vi "Dymin_FPGA_Main.vi"() -> ()   [LabVIEW 2016]
doc: "This VI demonstrates how to use an external signal to control the execution rate of a while loop."
uses:
  <vilib>/Platform/TimedLoop/XDataNode/timing_clust.ctl
  <vilib>/Platform/TimedLoop/XDataNode/nitl_modes.ctl
  <vilib>/Platform/TimedLoop/XDataNode/wakeup.ctl
  <vilib>/rvi/Emulation/niFpgaGetClockAttributes.vi
  <vilib>/rvi/Emulation/niFpgaSctlEmulationGetInTimedLoop.vi
  <vilib>/rvi/Emulation/niFpgaEmulationReportErrorSimple.vi
  <vilib>/rvi/eio/common/nirviEmuTemplateMethod_errors.vi
  <vilib>/rvi/Emulation/niFpgaCriticalErrorInLSC.vi
  <vilib>/rvi/DataTransferAndStorage/Container/Common/niFpgaContainerExecOnDevCompGetState.vi
  <vilib>/rvi/Emulation/niFpgaEmulationIsFPGAContextNoSignature.vi
  <vilib>/rvi/errors/niFpgaSetErrorForExecOnDevCompSimple.vi
  <vilib>/rvi/eio/common/nirviEmuReportErrorAndStop.vi
  <vilib>/rvi/DataTransferAndStorage/Container/Common/niFpgaContainerGetUniqueNameForEmu.vi
  <vilib>/rvi/FIFO/Fifo_Resource/nirvififoEmulationSetSize.vi
  <vilib>/rvi/FIFO/Fifo_Resource/nirviFifoEmulationQueueMgr.vi
  <instcachedir>/0/nirviFifoEmulationQueueMgr_E5CAEC123FF24DC58D834DCA3CDAA9B5.lvgen/nirviFifoEmulationQueueMgr_E5CAEC123FF24DC58D834DCA3CDAA9B5_001.vi
  <vilib>/rvi/FIFO/Fifo_Resource/nirvififoEmulationDetermineInputValidOut.vi
  <vilib>/rvi/FIFO/Fifo_Resource/nirvififoEmulationCreateLock.vi
  <vilib>/rvi/Emulation/niFpgaProcessEmulError.vi
  <vilib>/rvi/FIFO/Fifo_Resource/nirvififoEmulationObtainLock.vi
  <vilib>/rvi/FIFO/Fifo_Resource/nirvififoEmulationReleaseLock.vi
  <vilib>/rvi/occurrence/nirviWaitOnOccurrenceBase.vi
  <vilib>/rvi/errors/nirviReportUnexpectedCaseInternalError.vi
  <vilib>/rvi/errors/nirviReportUnexpectedCaseInternalError (U32).vi
  <vilib>/Utility/error.llb/Clear Errors.vi
  <vilib>/rvi/interface/RandomDataEmulation/niFpgaRandomDataHandleErrors.vi
  <vilib>/eio/EIONode/EIONode.xnode
  <vilib>/Platform/TimedLoop/XDataNode/XDataNode.xnode
  <vilib>/rvi/DataTransferAndStorage/Container/XNode/niFpgaContainer.xnode
  <vilib>/rvi/FIFO/Fifo_Resource/niFpgaFifoEmulationRefIn.vi
  <vilib>/Platform/TimedLoop/XDataNode/XDNodeRunTimeDep.lvlib
panel:
  in  "Dymin On?":bool
  in  "stop 4":bool
  in  "stop 3":bool
  in  "stop 2":bool
  in  "stop":bool
  out "Index":i32
  out "Dymin Step":i32
  out "Counts":i32
  out "Last Index":i32
  out "Last Counts":i32
  in  "Time (#80MHz periods)":i32[](array[numeric])=[32, 32, 32, 32]
  in  "Threshold (counts)":i32[](array[numeric])=[0, 0, 0, 0]
  in  "AOM Volts":u16[](array[numeric])=[0, 82, 164, 246]
  # "12 bit ADC volts"
  # ".1=82\n.2=164\n.3=246"
  # "16=200ns\n32=400ns"
  # "0 value means the step before it was the last step"
  # "v5 new settings for multiplexer\nv6 new DIOs on 9/24/2020\nv7 new DIOs on 11/24/2020\nv8_2 Dymin on button"
  # "step with Time_i=0 is not done, last step must have a time and first step with time 0 is \nOR find another way to finish the Dymin, but for now do it this way."
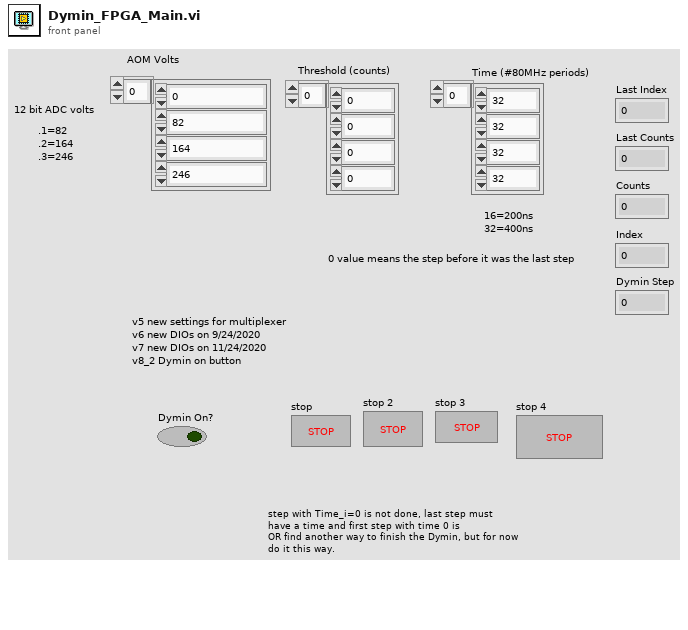
[diagram p1: front panel]
types:
  T1 = typedef "XDNodeRunTimeDep.lvlib/timing_clust.ctl" = cluster{"Expected End [f-1]":u64, "Actual End [f-1]":u64, "Finished Late? [f-1]":bool, "Expected End [i-1]":u64, "Actual End [i-1]":u64, "Finished Late? [i-1]":bool, "Expected Start [i]":u64, "Actual Start [i]":u64, "Expected Start [f]":u64, "Actual Start [f]":u64, "Source Name":string, "Structure Name":string, "Period":i64, "Deadline":i64, "Offset":i64, "Start":i64, "Priority":i32, "Timeout":i32, "Mode":T2, "Wakeup Reason":T3, "Error":errorcluster, "Source Type":string, "Secondary Source Type":string, "Global End Time":u64, "Global Start Time":u64, "Frame Duration":u64, "Iteration Duration":u64, "Assigned CPU":i32, "I/O Scan Engine Mode":u32}
  T2 = typedef "XDNodeRunTimeDep.lvlib/nitl_modes.ctl" = enum32{"No Change", "Process missed periods, maintain original phase", "Discard missed periods, maintain original phase", "Process missed periods, ignore original phase", "Discard missed periods, ignore original phase"}
  T3 = typedef "XDNodeRunTimeDep.lvlib/wakeup.ctl" = enum32{"Normal", "Aborted", "Asynchronous wakeup", "Timing source error", "Timed loop error", "Timeout"}
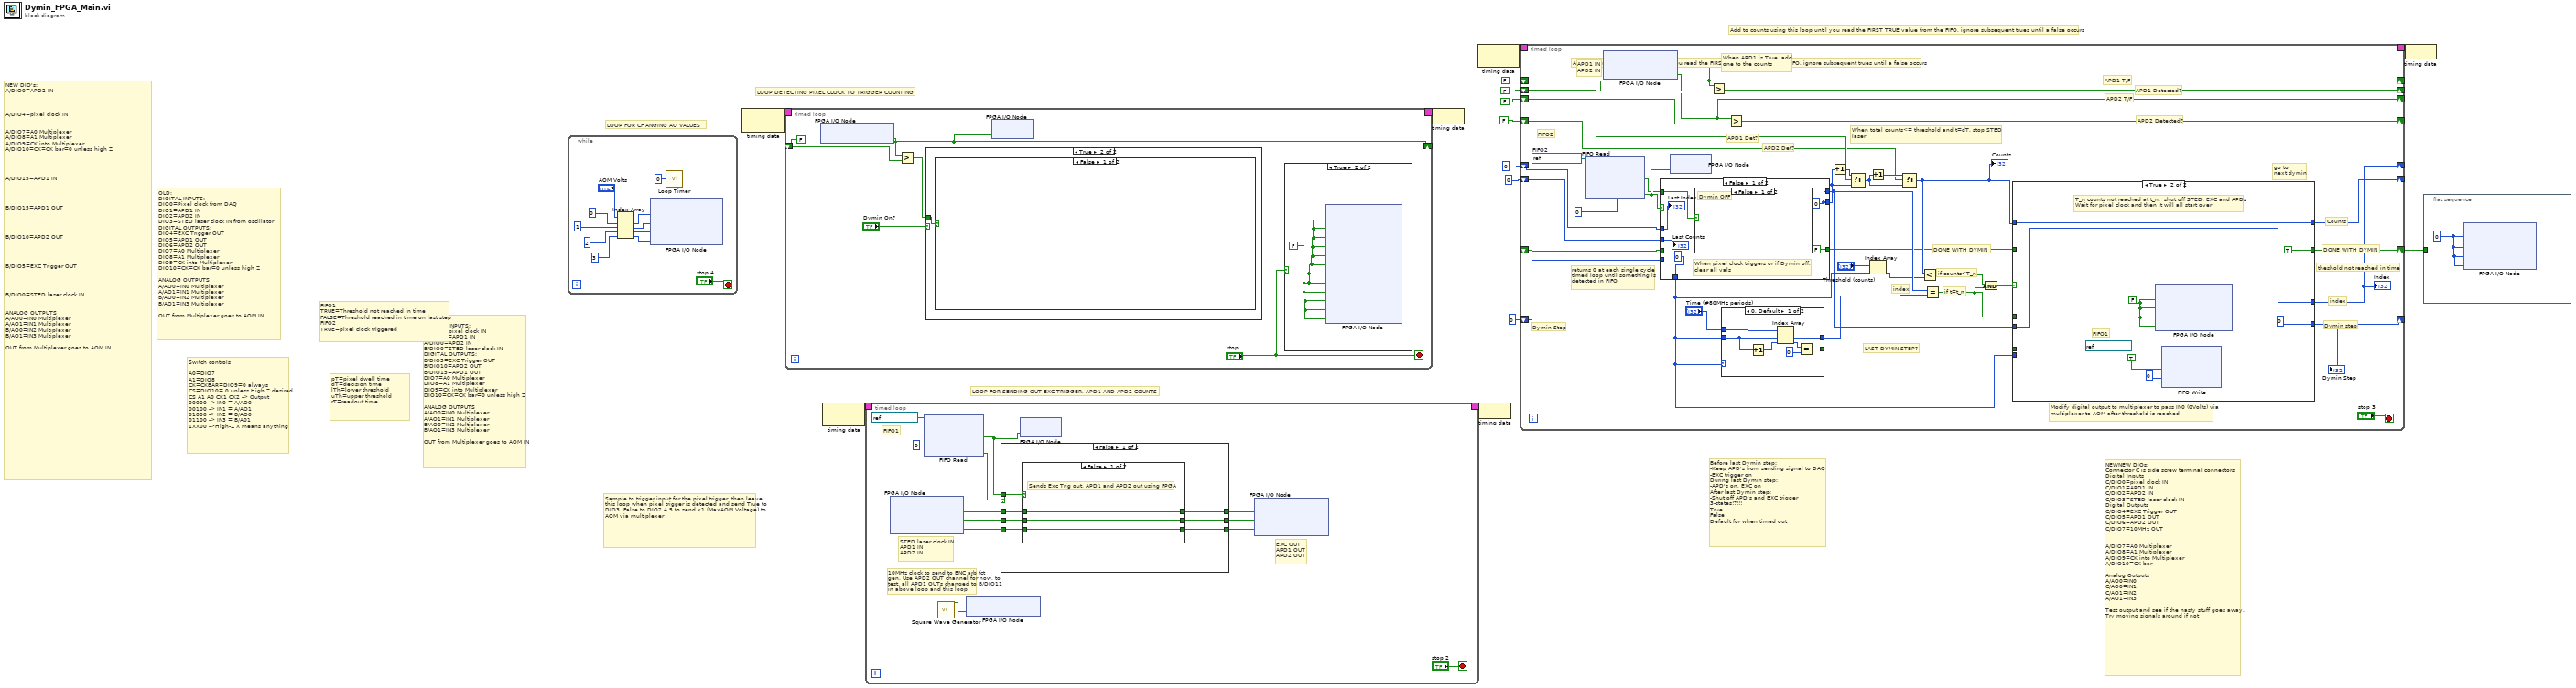
[diagram p0: block diagram]
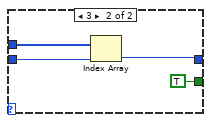
[diagram p2: hidden frame]
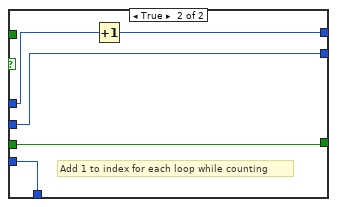
[diagram p4: hidden frame]
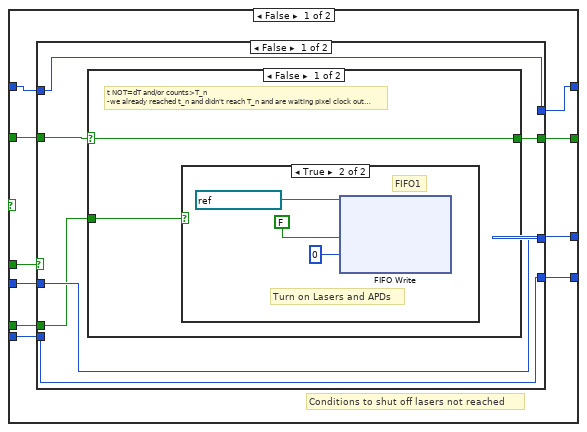
[diagram p5: hidden frame]
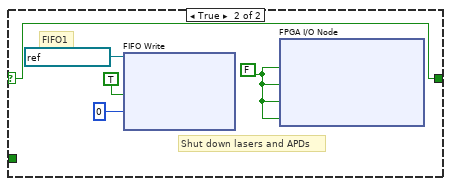
[diagram p7: hidden frame]
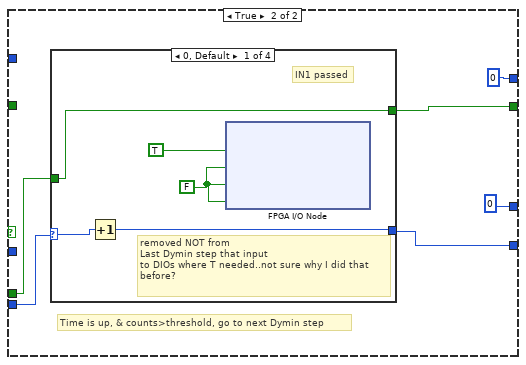
[diagram p8: hidden frame]
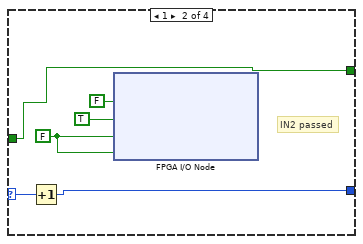
[diagram p9: hidden frame]
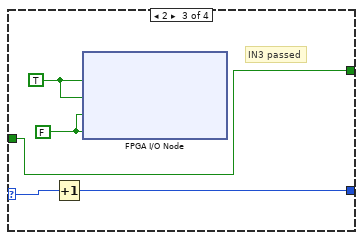
[diagram p10: hidden frame]
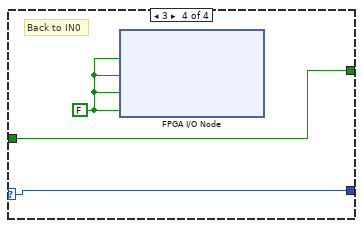
[diagram p11: hidden frame]
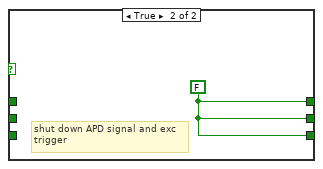
[diagram p12: hidden frame]
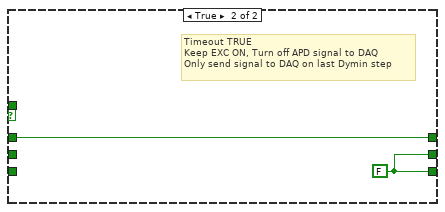
[diagram p13: hidden frame]
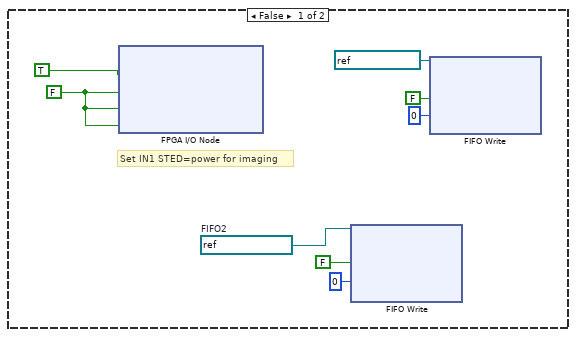
[diagram p14: hidden frame]
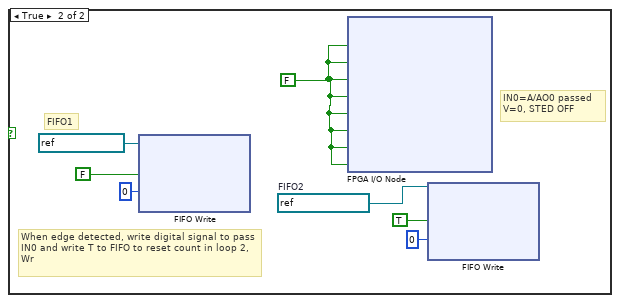
[diagram p15: hidden frame]
diagram:
  # "LOOP FOR CHANGING AO VALUES"
  # "NEWNEW DIOs:\nConnector C is side screw terminal connectors\nDigital Inputs\nC/DIO0=pixel clock IN\nC/DIO1=APD1 IN\nC/DIO2=APD2 IN\nC/DIO3=STED laser clock IN\nDigital Outputs\nC/DIO4=EXC Trigger OUT\nC/DIO5=APD1 OUT\nC/DIO6=APD2 OUT\nC/DIO7=10MHz OUT\n\n \nA/DIO7=A0 Multiplexer\nA/DIO8=A1 Multiplexer\nA/DIO9=CK into Multiplexer\nA/DIO10=CK bar\n\nAnalog Outputs\nA/AO0=IN0\nC/AO0=IN1\nC/AO1=IN2\nA/AO1=IN3\n\nTest output and see if the nasty stuff goes away.\nTry moving signals around if not"
  # "NEW DIO's:\nA/DIO0=APD2 IN\n\n\n\nA/DIO4=pixel clock IN\n\n\nA/DIO7=A0 Multiplexer\nA/DIO8=A1 Multiplexer\nA/DIO9=CK into Multiplexer\nA/DIO10=CK=CK bar=0 unless high Z\n\n\n\n\nA/DIO15=APD1 IN \n\n\n\n\nB/DIO15=APD1 OUT \n\n\n\n\nB/DIO10=APD2 OUT \n\n\n\n\nB/DIO5=EXC Trigger OUT\n\n\n\n\nB/DIO0=STED laser clock IN\n\n\nANALOG OUTPUTS\nA/AO0=IN0 Multiplexer\nA/AO1=IN1 Multiplexer\nB/AO0=IN2 Multiplexer\nB/AO1=IN3 Multiplexer\n\nOUT from Multiplexer goes to AOM IN"
  # "NEW:\nDIGITAL INPUTS:\nA/DIO4=pixel clock IN\nA/DIO15=APD1 IN \nA/DIO0=APD2 IN\nB/DIO0=STED laser clock IN\nDIGITAL OUTPUTS:\nB/DIO5=EXC Trigger OUT\nB/DIO10=APD2 OUT\nB/DIO15=APD1 OUT\nDIO7=A0 Multiplexer\nDIO8=A1 Multiplexer\nDIO9=CK into Multiplexer\nDIO10=CK=CK bar=0 unless high Z\n\nANALOG OUTPUTS\nA/AO0=IN0 Multiplexer\nA/AO1=IN1 Multiplexer\nB/AO0=IN2 Multiplexer\nB/AO1=IN3 Multiplexer\n\nOUT from Multiplexer goes to AOM IN"
  # "Switch controls\n\nA0=DIO7\nA1=DIO8\nCK=CKBAR=DIO9=0 always\nCS=DIO10= 0 unless High Z desired\nCS A1 A0 CK1 CK2 -> Output\n00000 -> IN0 = A/AO0\n00100 -> IN1 = A/AO1\n01000 -> IN2 = B/AO0\n01100 -> IN3 = B/A01\n1XX00 ->High-Z X means anything"
  # "FIFO1\nTRUE=Threshold not reached in time\nFALSE=Threshold reached in time on last step\nFIFO2\nTRUE=pixel clock triggered"
  # "OLD:\nDIGITAL INPUTS:\nDIO0=Pixel clock from DAQ\nDIO1=APD1 IN \nDIO2=APD2 IN\nDIO3=STED laser clock IN from oscillator\nDIGITAL OUTPUTS:\nDIO4=EXC Trigger OUT\nDIO5=APD1 OUT\nDIO6=APD2 OUT\nDIO7=A0 Multiplexer\nDIO8=A1 Multiplexer\nDIO9=CK into Multiplexer\nDIO10=CK=CK bar=0 unless high Z\n\nANALOG OUTPUTS\nA/AO0=IN0 Multiplexer\nA/AO1=IN1 Multiplexer\nB/AO0=IN2 Multiplexer\nB/AO1=IN3 Multiplexer\n\nOUT from Multiplexer goes to AOM IN"
  # "Before last Dymin step:\n-Keep APD's from sending signal to DAQ\n-EXC trigger on\nDuring last Dymin step:\n-APD's on, EXC on\nAfter last Dymin step:\n-Shut off APD's and EXC trigger\n3-states!?!!!\nTrue\nFalse\nDefault for when timed out"
  # "Add to counts using this loop until you read the FIRST TRUE value from the FIFO, ignore subsequent trues until a false occurs"
  # "LOOP FOR SENDING OUT EXC TRIGGER, APD1 AND APD2 COUNTS"
  # "LOOP DETECTING PIXEL CLOCK TO TRIGGER COUNTING"
  # "Add to counts using this loop until you read the FIRST TRUE value from the FIFO, ignore subsequent trues until a false occurs"
  # "Sample to trigger input for the pixel trigger, then leave this loop when pixel trigger is detected and send True to DIO3, False to DIO2,4,5 to send x1 (MaxAOM Voltage) to AOM via multiplexer"
  # "pT=pixel dwell time\ndT=decision time\nlTh=lower threshold\nuTh=upper threshold\nrT=readout time"
  n1 = while {
    stop <- "stop 4" stop-if-true
    n2 = Index Array(array="AOM Volts", index #1=0 ("index"), index #2=1 ("index"), index #3=2 ("index"), index #4=3 ("index")) -> (element #1=w21:u16, element #2=w17:u16, element #3=w16:u16, element #4=w18:u16)
    n3 = xnode "FPGA I/O Node"("ConnectorA/AO0"=w21, "ConnectorC/AO0"=w17, "ConnectorC/AO1"=w16, "ConnectorA/AO1"=w18) -> ()  [unwired: 4 in, 4 out]
    n4 = call "Loop Timer"("Count(mSec)"=u32 0) -> ()  [unwired: 1 out]
  }
  n5 = node-c288() -> (w15:T1)  [unwired: 1 in]
  n6 = timed-loop {
    timing: w15 -> [_]
    timing-out: [_] -> w14
    shift-right: [w28] -> _
    shift-left: FALSE -> [w31]
    stop <- "stop" stop-if-true
    n7 = xnode "FPGA I/O Node"() -> ("ConnectorC/DIO0"=w28:bool)  [unwired: 1 in, 1 out]
    n8 = Greater?(x=w28, y=w31) -> (0:w30:bool)
    n9 = case shown="True" "Dymin On?" {
      tunnel: w30 -> [_ w40]
      frame False {
        w34 = refnum<k21> "A.DO1 DMA"  # FIFO2
        w35 = FALSE ("ConnectorA/DIO8")
        # "Set IN1 STED=power for imaging"
        n10 = xnode "FPGA I/O Node"("ConnectorA/DIO7"=TRUE, "ConnectorA/DIO8"=w35, "ConnectorA/DIO9"=w35, "ConnectorA/DIO10"=w35) -> ()  [unwired: 4 in, 4 out]
        n11 = xnode ("FIFO Write")("Element"=FALSE, "Timeout"=0, "FIFO In"=w34) -> ()  [unwired: 2 out]
        n12 = xnode ("FIFO Write")("Element"=FALSE, "Timeout"=0, "FIFO In"=refnum<k21> "A.DI0 DMA") -> ()  [unwired: 2 out]
      }
      frame True {
        n13 = case shown="False" w40 {
          frame False {
          }
          frame True {
            w41 = FALSE ("ConnectorA/DIO4")
            w47 = refnum<k21> "A.DO1 DMA"  # FIFO2
            # "FIFO1"
            # "When edge detected, write digital signal to pass IN0 and write T to FIFO to reset count in loop 2, Wr"
            # "IN0=A/AO0 passed\nV=0, STED OFF"
            n14 = xnode ("FIFO Write")("Element"=FALSE, "Timeout"=0, "FIFO In"=refnum<k21> "A.DI0 DMA") -> ()  [unwired: 2 out]
            n15 = xnode "FPGA I/O Node"("ConnectorC/DIO4"=w41, "ConnectorC/DIO5"=w41, "ConnectorC/DIO6"=w41, "ConnectorC/DIO7"=w41, "ConnectorA/DIO7"=w41, "ConnectorA/DIO8"=w41, "ConnectorA/DIO9"=w41, "ConnectorA/DIO10"=w41) -> ()  [unwired: 8 in, 8 out]
            n16 = xnode ("FIFO Write")("Element"=TRUE, "Timeout"=0, "FIFO In"=w47) -> ()  [unwired: 2 out]
          }
        }
      }
    }
    n17 = xnode "FPGA I/O Node"("LED0"=w28) -> ()  [unwired: 1 in, 1 out]
    n18 = case shown="True" "stop" {
      frame False {
      }
      frame True {
        w48 = FALSE
        n19 = xnode "FPGA I/O Node"("ConnectorC/DIO0"=w48, "ConnectorC/DIO1"=w48, "ConnectorC/DIO2"=w48, "ConnectorC/DIO3"=w48, "ConnectorC/DIO4"=w48, "ConnectorC/DIO5"=w48, "ConnectorC/DIO6"=w48, "ConnectorC/DIO7"=w48, "ConnectorA/DIO7"=w48, "ConnectorA/DIO8"=w48, "ConnectorA/DIO9"=w48, "ConnectorA/DIO10"=w48) -> ()  [unwired: 12 in, 12 out]
      }
    }
  }
  n20 = node-c288() -> (w12:T1)  [unwired: 1 in]
  n21 = timed-loop {
    timing: w12 -> [_]
    timing-out: [_] -> w11
    stop <- "stop 2" stop-if-true
    # "10MHz clock to send to BNC arb fct gen, Use APD2 OUT channel for now, to test, all APD1 OUTs changed to B/DIO11 in above loop and this loop"
    # "EXC OUT\nAPD1 OUT\nAPD2 OUT"
    # "FIFO1"
    # "STED laser clock IN\nAPD1 IN\nAPD2 IN"
    n22 = xnode "FPGA I/O Node"() -> ("ConnectorC/DIO3"=w60:bool, "ConnectorC/DIO1"=w58:bool, "ConnectorC/DIO2"=w57:bool)  [unwired: 3 in, 3 out]
    n23 = xnode ("FIFO Read")("Timeout"=0, "FIFO In"=refnum<k21> "A.DI0 DMA") -> ("Element"=w51:bool, "Timed Out?"=w54:bool)  [unwired: 1 out]
    n24 = call "Square Wave Generator"() -> ("square wave out"=w53:bool)  [unwired: 15 in]
    n25 = xnode "FPGA I/O Node"("ConnectorC/DIO7"=w53) -> ()  [unwired: 1 in, 1 out]
    n26 = case shown="False" w54 {
      tunnel: w60 -> [w69 w75]
      tunnel: w51 -> [w68 _]
      tunnel: [w67 w75] -> w59
      tunnel: w58 -> [w66 _]
      tunnel: w57 -> [w65 _]
      tunnel: [w64 w74] -> w56
      tunnel: [w63 w74] -> w55
      frame False {
        n27 = case shown="False" w68 {
          tunnel: w69 -> [w72 _]
          tunnel: [w72 w73] -> w67
          tunnel: w66 -> [w71 _]
          tunnel: w65 -> [w70 _]
          tunnel: [w71 w73] -> w64
          tunnel: [w70 w73] -> w63
          frame False {
            # "Sends Exc Trig out, APD1 and APD2 out using FPGA"
          }
          frame True {
            w73 = FALSE ("ConnectorA/DIO3")
            # "shut down APD signal and exc trigger"
          }
        }
      }
      frame True {
        w74 = FALSE
        # "Timeout TRUE\nKeep EXC ON, Turn off APD signal to DAQ\nOnly send signal to DAQ on last Dymin step"
      }
    }
    n28 = xnode "FPGA I/O Node"("LED2"=w51) -> ()  [unwired: 1 in, 1 out]
    n29 = xnode "FPGA I/O Node"("ConnectorC/DIO4"=w59, "ConnectorC/DIO5"=w56, "ConnectorC/DIO6"=w55) -> ()  [unwired: 3 in, 3 out]
  }
  n30 = node-c288(w14) -> ()
  n31 = node-c288() -> (w10:T1)  [unwired: 1 in]
  n32 = node-c288(w11) -> ()
  n33 = timed-loop {
    timing: w10 -> [_]
    timing-out: [_] -> w9
    shift-right: [w112] -> _
    shift-left: FALSE -> [w114]
    shift-right: [w107] -> _
    shift-left: FALSE -> [w102]
    shift-right: [w96] -> _
    shift-left: 0 -> [w109]
    shift-right: [w91] -> _
    shift-left: FALSE -> [w103]
    shift-right: [w108] -> _
    shift-left: FALSE -> [w106]
    shift-right: [w92] -> _
    shift-left: 0 -> [w104]
    shift-right: [w98] -> _
    shift-left: 0 -> [w82]
    shift-right: [w86] -> w1
    shift-left: _ -> [w84]
    stop <- "stop 3" stop-if-true
    w95 = refnum<k21> "A.DO1 DMA"  # FIFO2
    # "APD1 IN\nAPD2 IN"
    # "DONE WITH DYMIN"
    # "go to\nnext dymin"
    # "DONE WITH DYMIN"
    # "LAST DYMIN STEP?"
    # "theshold not reached in time"
    # "Dymin Step"
    # "Dymin step"
    # "FIFO2"
    # "if counts<T_n"
    # "if t=t_n"
    # "returns 0 at each single cycle timed loop until something is detected in FIFO"
    # "Modify digital output to multiplexer to pass IN0 (0Volts) via multiplexer to AOM after threshold is reached"
    # "When total counts<= threshold and t=dT, stop STED laser"
    # "index"
    # "APD1 Det?"
    # "APD2 Det?"
    # "APD2 Detected?"
    # "APD2 T/F"
    # "APD1 Detected?"
    # "APD1 T/F"
    # "index"
    # "Counts"
    # "When APD1 is True, add one to the counts"
    n34 = xnode ("FIFO Read")("Timeout"=0, "FIFO In"=w95) -> ("Element"=w78:bool, "Timed Out?"=w79:bool)  [unwired: 1 out]
    n35 = xnode "FPGA I/O Node"() -> ("ConnectorC/DIO1"=w112:bool, "ConnectorC/DIO2"=w108:bool)  [unwired: 2 in, 2 out]
    n36 = case shown="False" w79 {
      tunnel: [w130 w134] -> w110
      tunnel: [w130 w135] -> w97
      tunnel: w109 -> [w131 w136]
      tunnel: w104 -> [w129 w134]
      tunnel: w84 -> [_ w133]
      tunnel: [FALSE w133] -> w83
      tunnel: w82 -> [_ w132]
      tunnel: [0 w132] -> w81
      tunnel: w78 -> [w126 _]
      frame False {
        w130 = 0
        # "When pixel clock triggers or if Dymin off, \nclear all vals"
        n37 = case shown="False" w126 {
          frame False {
            # "Dymin OFF"
          }
          frame True {
            # "Dymin ON"
          }
        }
        "Last Index" <- w131
        "Last Counts" <- w129
      }
      frame True {
        # "Add 1 to index for each loop while counting"
        n38 = Increment(x=w136) -> (x+1=w135:i32)
      }
    }
    n39 = xnode "FPGA I/O Node"("LED1"=w79) -> ()  [unwired: 1 in, 1 out]
    n40 = Greater?(x=w112, y=w114) -> (0:w91:bool)
    n41 = case shown="0, Default" w81 {
      tunnel: [w121 w123] -> w90
      tunnel: w81 -> [w119 w124]
      tunnel: [w116 TRUE] -> w88
      tunnel: "Time (#80MHz periods)" -> [w115 w125]
      frame 0, Default {
        n42 = Increment(x=w119) -> (x+1=w120:i32)
        n43 = Index Array(array=w115, index #1=w119, index #2=w120) -> (element #1=w121:i32, element #2=w118:i32)
        n44 = Equal?(x=w118, y=0) -> (x = y?=w116:bool)
      }
      frame 3 {
        n45 = Index Array(array=w125, index=w124) -> (element=w123:i32)
      }
    }
    n46 = Greater?(x=w108, y=w106) -> (0:w107:bool)
    n47 = Increment(x=w110) -> (x+1=w113:i32)
    n48 = Select(t=w113, s=w103, f=w110) -> (s? t:f=w99:i32)
    n49 = Index Array(array="Threshold (counts)", index=w81) -> (element=w89:i32)
    n50 = Increment(x=w99) -> (x+1=w105:i32)
    n51 = Select(t=w105, s=w102, f=w99) -> (s? t:f=w93:i32)
    "Counts" <- w93
    n52 = Less?(x=w93, y=w89) -> (x < y?=w101:bool)
    n53 = Equal?(x=w97, y=w90) -> (x = y?=w87:bool)
    n54 = And(x=w101, y=w87) -> (x .and. y?=w100:bool)
    n55 = case shown="True" w100 {
      tunnel: w81 -> [w146 _]
      tunnel: [w145 0] -> w98
      tunnel: w97 -> [w144 w192]
      tunnel: [w143 w192] -> w96
      tunnel: w93 -> [w141 w190]
      tunnel: [w142 w190] -> w92
      tunnel: w88 -> [w140 _]
      tunnel: w87 -> [w139 _]
      tunnel: [w138 TRUE] -> w86
      tunnel: w83 -> [w137 _]
      frame False {
        # "Conditions to shut off lasers not reached"
        n56 = case shown="False" w139 {
          tunnel: w146 -> [w152 w166]
          tunnel: [w152 w165] -> w145
          tunnel: w144 -> [w151 _]
          tunnel: [w151 0] -> w143
          tunnel: [w150 0] -> w142
          tunnel: w141 -> [w150 _]
          tunnel: w140 -> [w147 w164]
          tunnel: [w149 w163] -> w138
          tunnel: w137 -> [w148 _]
          frame False {
            # "t NOT=dT and/or counts>T_n\n-we already reached t_n and didn't reach T_n and are waiting pixel clock out\n-we haven't reached t_n and are waiting\n-"
            n57 = case shown="False" w148 {
              selector: w148 -> [w154 w158]
              tunnel: [w154 w158] -> w149
              tunnel: w147 -> [w153 _]
              frame False {
                n58 = case shown="True" w153 {
                  frame False {
                  }
                  frame True {
                    # "Turn on Lasers and APDs"
                    # "FIFO1"
                    n59 = xnode ("FIFO Write")("Element"=FALSE, "Timeout"=0, "FIFO In"=refnum<k21> "A.DI0 DMA") -> ()  [unwired: 2 out]
                  }
                }
              }
              frame True {
                w159 = FALSE
                # "Shut down lasers and APDs"
                # "FIFO1"
                n60 = xnode ("FIFO Write")("Element"=TRUE, "Timeout"=0, "FIFO In"=refnum<k21> "A.DI0 DMA") -> ()  [unwired: 2 out]
                n61 = xnode "FPGA I/O Node"("ConnectorA/DIO7"=w159, "ConnectorA/DIO8"=w159, "ConnectorA/DIO9"=w159, "ConnectorA/DIO10"=w159) -> ()  [unwired: 4 in, 4 out]
              }
            }
          }
          frame True {
            # "Time is up, & counts>threshold, go to next Dymin step"
            n62 = case shown="0, Default" w166 {
              selector: w166 -> [w173 w179 w184 w185]
              tunnel: [w172 w178 w183 w185] -> w165
              tunnel: w164 -> [w170 w176 w182 w186]
              tunnel: [w170 w176 w182 w186] -> w163
              frame 0, Default {
                w171 = FALSE ("ConnectorA/DIO4")
                # "removed NOT from\nLast Dymin step that input\nto DIOs where T needed..not sure why I did that\nbefore?"
                # "IN1 passed"
                n63 = Increment(x=w173) -> (x+1=w172:i32)
                n64 = xnode "FPGA I/O Node"("ConnectorA/DIO7"=TRUE, "ConnectorA/DIO8"=w171, "ConnectorA/DIO9"=w171, "ConnectorA/DIO10"=w171) -> ()  [unwired: 4 in, 4 out]
              }
              frame 1 {
                w177 = FALSE ("ConnectorA/DIO4")
                # "IN2 passed"
                n65 = Increment(x=w179) -> (x+1=w178:i32)
                n66 = xnode "FPGA I/O Node"("ConnectorA/DIO7"=FALSE, "ConnectorA/DIO8"=TRUE, "ConnectorA/DIO9"=w177, "ConnectorA/DIO10"=w177) -> ()  [unwired: 4 in, 4 out]
              }
              frame 2 {
                w181 = TRUE ("ConnectorA/DIO7")
                w180 = FALSE ("ConnectorA/DIO4")
                # "IN3 passed"
                n67 = Increment(x=w184) -> (x+1=w183:i32)
                n68 = xnode "FPGA I/O Node"("ConnectorA/DIO7"=w181, "ConnectorA/DIO8"=w181, "ConnectorA/DIO9"=w180, "ConnectorA/DIO10"=w180) -> ()  [unwired: 4 in, 4 out]
              }
              frame 3 {
                w187 = FALSE ("ConnectorA/DIO4")
                # "Back to IN0"
                n69 = xnode "FPGA I/O Node"("ConnectorA/DIO7"=w187, "ConnectorA/DIO8"=w187, "ConnectorA/DIO9"=w187, "ConnectorA/DIO10"=w187) -> ()  [unwired: 4 in, 4 out]
              }
            }
          }
        }
      }
      frame True {
        w195 = FALSE
        # "T_n counts not reached at t_n,  shut off STED, EXC and APDs\nWait for pixel clock and then it will all start over"
        # "FIFO1"
        n70 = xnode "FPGA I/O Node"("ConnectorA/DIO7"=w195, "ConnectorA/DIO8"=w195, "ConnectorA/DIO9"=w195, "ConnectorA/DIO10"=w195) -> ()  [unwired: 4 in, 4 out]
        n71 = xnode ("FIFO Write")("Element"=TRUE, "Timeout"=0, "FIFO In"=refnum<k21> "A.DI0 DMA") -> ()  [unwired: 2 out]
      }
    }
    "Dymin Step" <- w98
    "Index" <- w96
  }
  n72 = node-c288(w9) -> ()
  n73 = flat-sequence {
    tunnel: w1 -> [_]
    frame #0 {
      w198 = u16 0 ("ConnectorA/AO0")
      n74 = xnode "FPGA I/O Node"("ConnectorA/AO0"=w198, "ConnectorA/AO1"=w198, "ConnectorC/AO0"=w198, "ConnectorC/AO1"=w198) -> ()  [unwired: 4 in, 4 out]
    }
  }
